vi "Encode JSON Recursive.vi"(4 "error in (no error)":errorcluster, 6 "String In":string, 7 "JSON Tree":variant) -> (0 "error out":errorcluster, 2 "String Out":string)   [LabVIEW 2011, in "i3-json.lvlib"]
uses:
  i3-json.lvlib
  JSON Types/JSON Type.ctl
  Generation Error.ctl
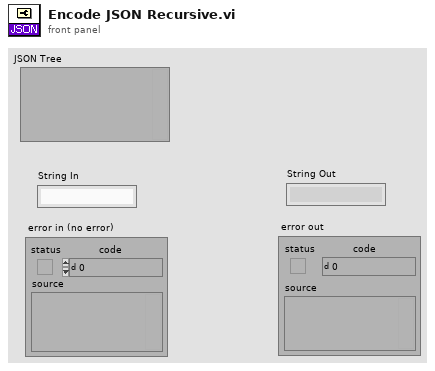
[diagram p1: front panel]
types:
  T1 = typedef "i3-json.lvlib/JSON Type.ctl" = enum8{"JSON Compatible", "JSON Array", "JSON Object", "JSON Null", "Double", "String", "Boolean", "Unknown"}
  T2 = typedef "i3-json.lvlib/Generation Error.ctl" = string
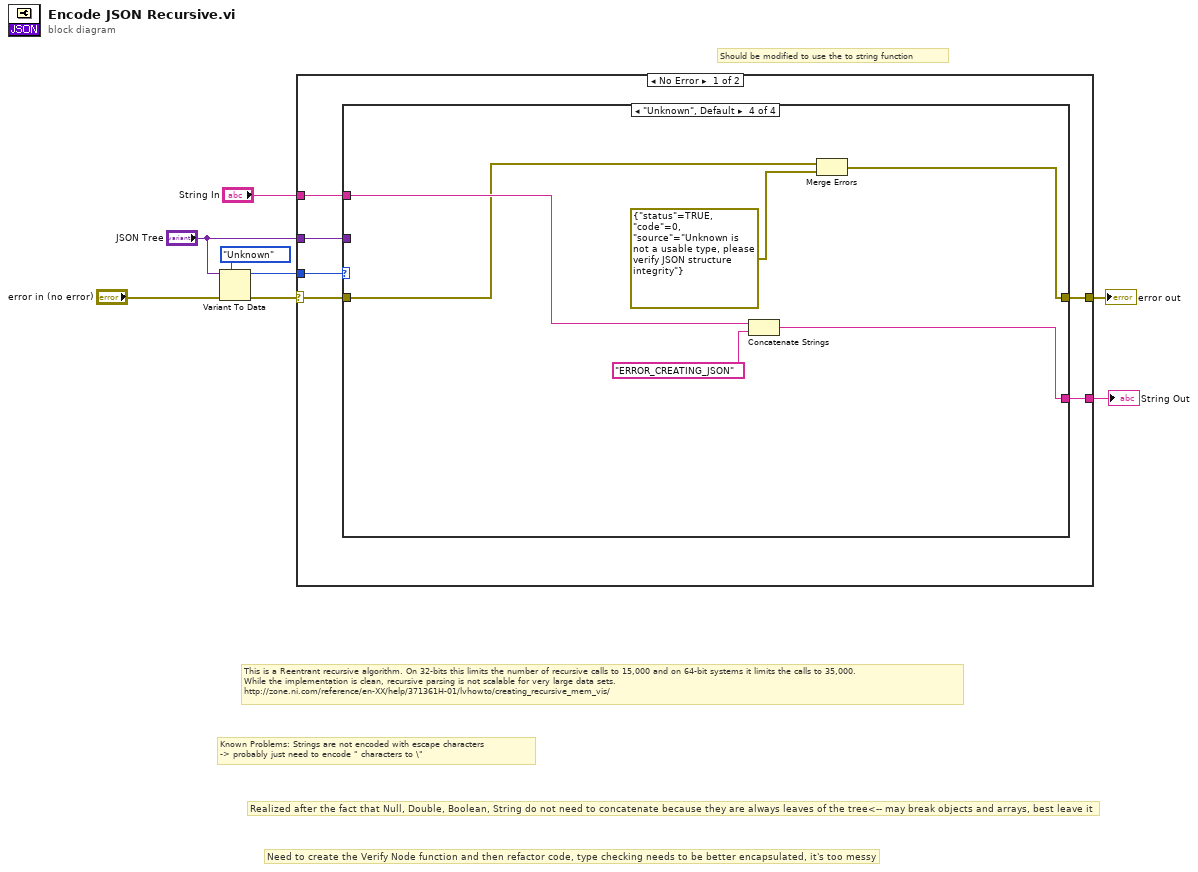
[diagram p0: block diagram]
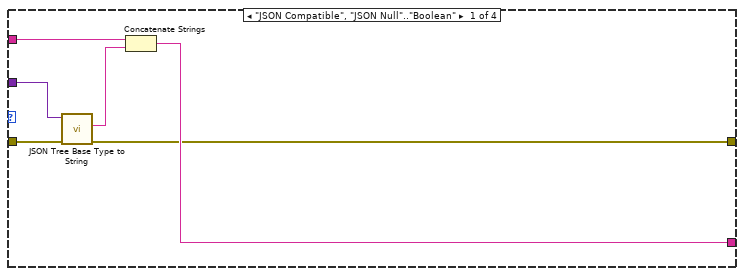
[diagram p2: hidden frame]
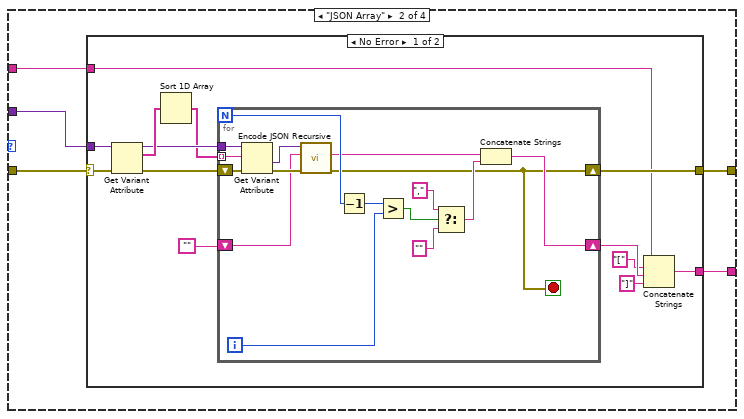
[diagram p3: hidden frame]
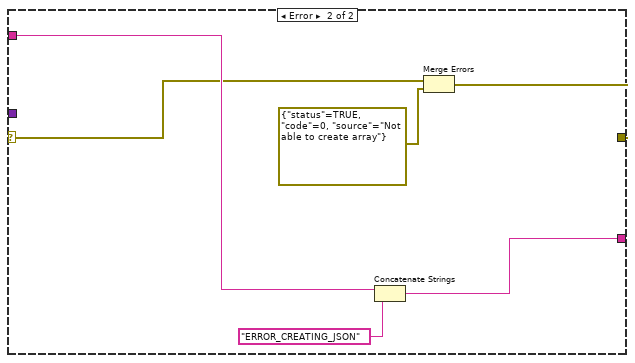
[diagram p4: hidden frame]
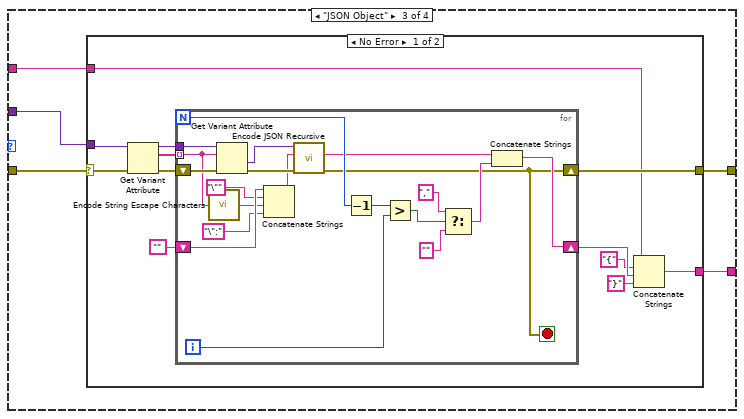
[diagram p5: hidden frame]
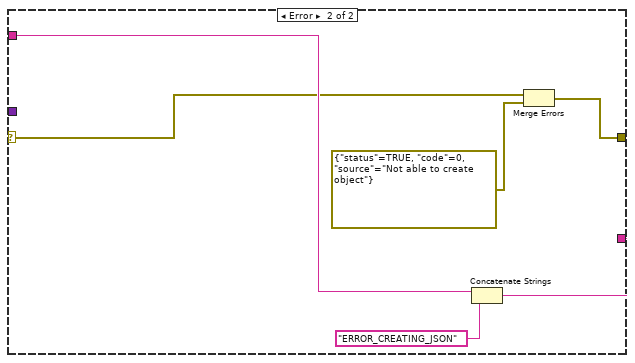
[diagram p6: hidden frame]
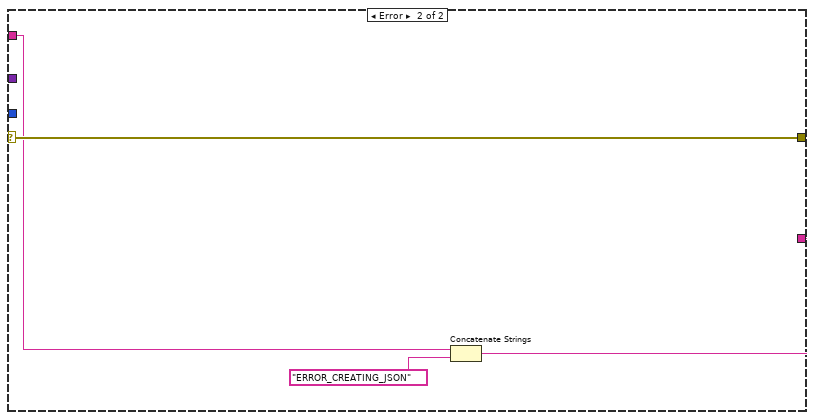
[diagram p7: hidden frame]
diagram:
  # "Should be modified to use the to string function"
  # "Need to create the Verify Node function and then refactor code, type checking needs to be better encapsulated, it's too messy"
  # "Realized after the fact that Null, Double, Boolean, String do not need to concatenate because they are always leaves of the tree<-- may break objects and arrays, best leave it"
  # "Known Problems: Strings are not encoded with escape characters\n-> probably just need to encode \" characters to \\\""
  # "This is a Reentrant recursive algorithm. On 32-bits this limits the number of recursive calls to 15,000 and on 64-bit systems it limits the calls to 35,000.\nWhile the implementation is clean, recursive parsing is not scalable for very large data sets.\nhttp://zone.ni.com/reference/en-XX/help/371361H-01/lvhowto/creating_recursive_mem_vis/"
  n1 = Variant To Data(error in="error in (no error)", type=JSON_Type."Unknown" ("JSON Type"), Variant="JSON Tree") -> (data=w5:T1, error out=w6:errorcluster)
  n2 = case shown="No Error" w6 {
    selector: w6 -> [w12 w113]
    tunnel: w5 -> [w14 _]
    tunnel: "JSON Tree" -> [w13 _]
    tunnel: "String In" -> [w11 w112]
    tunnel: [w10 w111] -> w2
    tunnel: [w9 w113] -> w1
    frame No Error {
      n3 = case shown="\"Unknown\", Default" w14 {
        tunnel: w13 -> [w15 w22 w65 _]
        tunnel: w12 -> [w16 w24 w61 w104]
        tunnel: w11 -> [w20 w23 w64 w108]
        tunnel: [w18 w21 w63 w107] -> w10
        tunnel: [w17 w25 w62 w106] -> w9
        frame "JSON Compatible", "JSON Null".."Boolean" {
          n4 = call "JSON Tree Base Type to String.vi"("error in (no error)"=w16, "JSON Tree Base Type"=w15) -> ("error out"=w17:errorcluster, "JSON Tree Base Type String"=w19:string)  [unwired: 8 in]
          n5 = Concatenate Strings(w20, w19) -> (w18:string)
        }
        frame "JSON Array" {
          n6 = case shown="No Error" w24 {
            selector: w24 -> [w37 w55]
            tunnel: [w32 w60] -> w25
            tunnel: w23 -> [w27 w59]
            tunnel: [w29 w57] -> w21
            tunnel: w22 -> [w38 _]
            frame No Error {
              n7 = Get Variant Attribute(Variant=w38, error in=w37) -> (duplicate Variant=w35:variant, names=w36:string[], error out=w34:errorcluster)  [unwired: 2 in, 1 out]
              n8 = Sort 1D Array(array=w36) -> (sorted array=w33:string[])
              n9 = for {
                N -> [w49]
                tunnel: w35 -> [w54]
                tunnel: w33 -> [w52] mode=indexing
                shift-right: [w39] -> w32
                shift-left: w34 -> [w53]
                shift-right: [w41] -> w31
                shift-left: "" -> [w40]
                i -> [w43]
                stop <- w39 stop-if-true
                n10 = Get Variant Attribute(Variant=w54, name=w52, error in=w53) -> (value=w50:variant, error out=w51:errorcluster)  [unwired: 1 in, 2 out]
                n11 = call "Encode JSON Recursive.vi"("error in (no error)"=w51, "String In"=w40, "JSON Tree"=w50) -> ("error out"=w39:errorcluster, "String Out"=w45:string)  [unwired: 3 in]
                n12 = Decrement(x=w49) -> (x-1=w42:i32)
                n13 = Greater?(x=w42, y=w43) -> (0:w48:bool)
                n14 = Select(t=",", s=w48, f="") -> (s? t:f=w44:string)
                n15 = Concatenate Strings(w45, w44) -> (w41:string)
              }
              n16 = Concatenate Strings(w27, "[" ("string"), w31, "]" ("string")) -> (w29:string)
            }
            frame Error {
              n17 = Concatenate Strings(w59, T2 "ERROR_CREATING_JSON" ("Generating Error")) -> (w57:string)
              n18 = Merge Errors(w55, errorcluster {"status"=TRUE, "code"=0, "source"="Not able to create array"} ("error in")) -> (w60:errorcluster)
            }
          }
        }
        frame "JSON Object" {
          n19 = case shown="No Error" w61 {
            selector: w61 -> [w76 w98]
            tunnel: [w73 w103] -> w62
            tunnel: w64 -> [w68 w102]
            tunnel: [w70 w100] -> w63
            tunnel: w65 -> [w77 _]
            frame No Error {
              n20 = Get Variant Attribute(Variant=w77, error in=w76) -> (duplicate Variant=w75:variant, names=w67:string[], error out=w74:errorcluster)  [unwired: 2 in, 1 out]
              n21 = for {
                N -> [w93]
                tunnel: w75 -> [w97]
                shift-right: [w80] -> w73
                shift-left: w74 -> [w96]
                shift-right: [w85] -> w72
                shift-left: "" -> [w84]
                tunnel: w67 -> [w78] mode=indexing
                i -> [w87]
                stop <- w80 stop-if-true
                n22 = call "Encode String Escape Characters.vi"("unescaped string in"=w78) -> ("escaped string out"=w79:string)
                n23 = Get Variant Attribute(Variant=w97, name=w78, error in=w96) -> (value=w94:variant, error out=w95:errorcluster)  [unwired: 1 in, 2 out]
                n24 = Concatenate Strings(w84, "\"" ("string"), w79, "\":" ("string")) -> (w81:string)
                n25 = call "Encode JSON Recursive.vi"("error in (no error)"=w95, "String In"=w81, "JSON Tree"=w94) -> ("error out"=w80:errorcluster, "String Out"=w89:string)  [unwired: 3 in]
                n26 = Decrement(x=w93) -> (x-1=w86:i32)
                n27 = Greater?(x=w86, y=w87) -> (0:w92:bool)
                n28 = Select(t=",", s=w92, f="") -> (s? t:f=w88:string)
                n29 = Concatenate Strings(w89, w88) -> (w85:string)
              }
              n30 = Concatenate Strings(w68, "{" ("string"), w72, "}" ("string")) -> (w70:string)
            }
            frame Error {
              n31 = Concatenate Strings(w102, T2 "ERROR_CREATING_JSON" ("Generating Error")) -> (w100:string)
              n32 = Merge Errors(w98, errorcluster {"status"=TRUE, "code"=0, "source"="Not able to create object"} ("error in")) -> (w103:errorcluster)
            }
          }
        }
        frame "Unknown", Default {
          n33 = Concatenate Strings(w108, T2 "ERROR_CREATING_JSON" ("Generating Error")) -> (w107:string)
          n34 = Merge Errors(w104, errorcluster {"status"=TRUE, "code"=0, "source"="Unknown is not a usable type, please verify JSON structure integrity"} ("error in")) -> (w106:errorcluster)
        }
      }
    }
    frame Error {
      n35 = Concatenate Strings(w112, T2 "ERROR_CREATING_JSON" ("string")) -> (w111:string)
    }
  }
  "String Out" <- w2
  "error out" <- w1
